vi "扫码枪设置.vi"() -> (2 "确定":bool)   [LabVIEW 2020]
uses:
  Global.vi
  <vilib>/Utility/config.llb/Write Key (String).vi
  <vilib>/Utility/config.llb/NI_LVConfig.lvlib
panel:
  in  "VISA资源名称":refnum<visa-resource-name>="COM5"
  out "error out":errorcluster caption="错误输出"
  in  "error in":errorcluster caption="错误输入（无错误）"
  in  "取消":bool
  in  "连接":bool
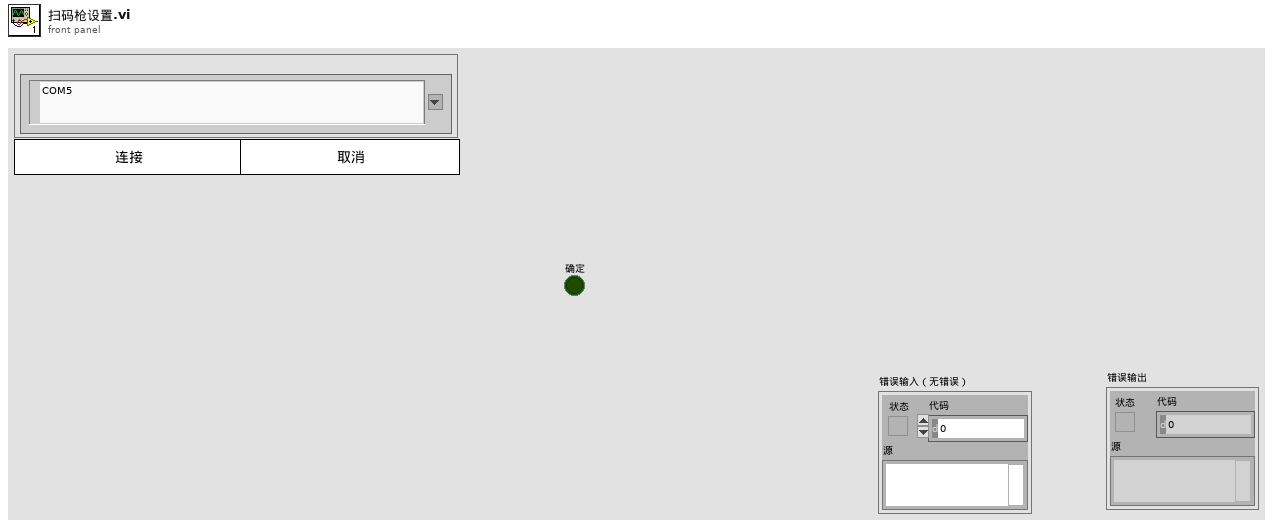
[diagram p1: front panel]
types:
  T1 = typedef "NI_LVConfig.lvlib/Config Data RefNum.ctl" = refnum<k1>
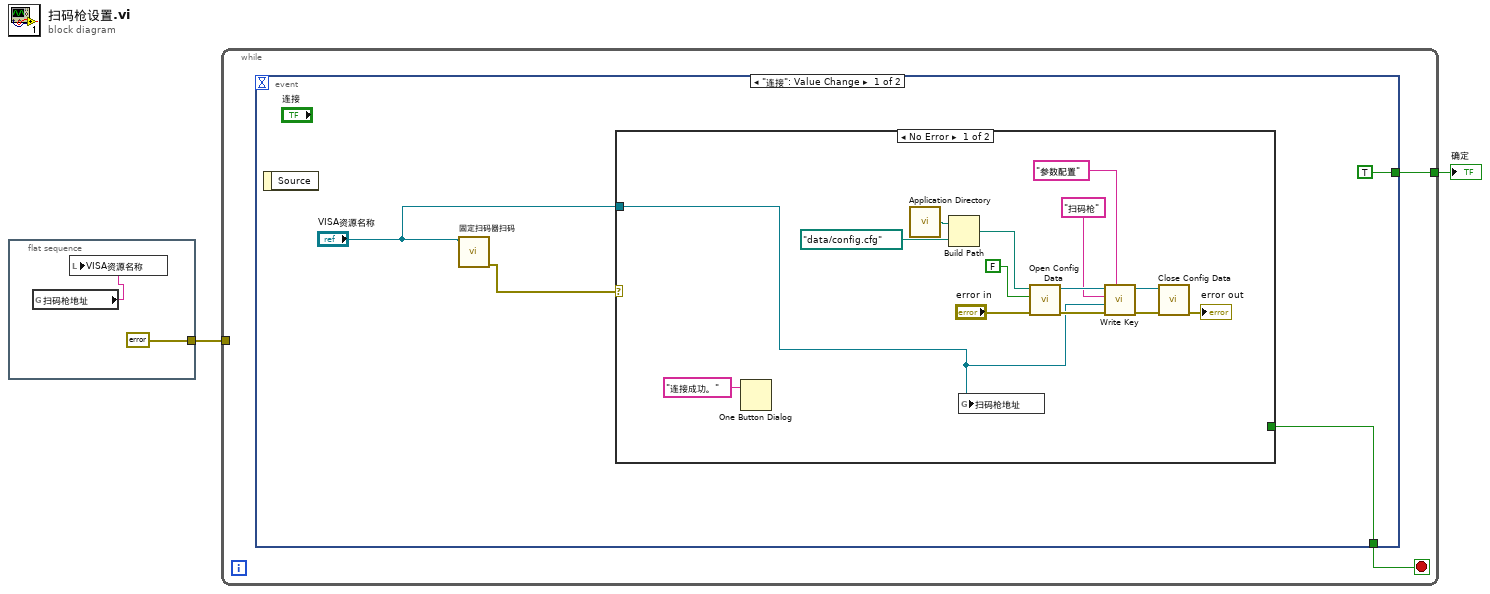
[diagram p0: block diagram]
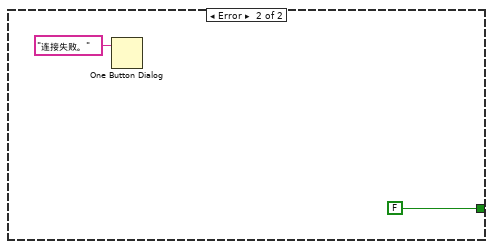
[diagram p2: hidden frame]
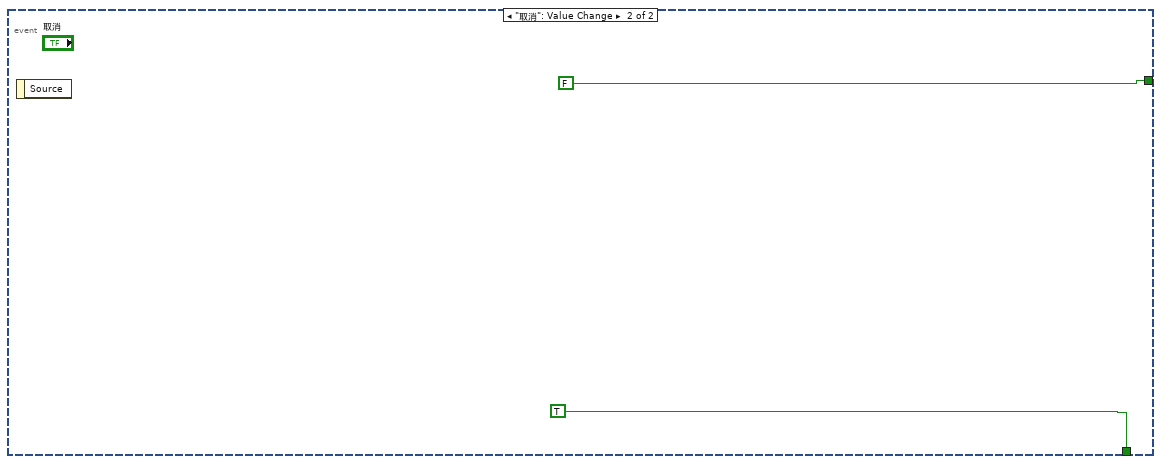
[diagram p3: hidden frame]
diagram:
  n1 = flat-sequence {
    tunnel: [errorcluster {"status"=FALSE, "code"=0, "source"=""} ("错误常量")] -> w1
    frame #0 {
      n2 = global read "Global.vi" "扫码枪地址"() -> (w3:string)
      n3 = local write "VISA资源名称"(w3) -> ()
    }
  }
  n4 = while {
    tunnel: [w5] -> w2
    tunnel: w1 -> [_]
    stop <- w6 stop-if-true
    n5 = event shown="[0] \"连接\": Value Change" {
      selector: _ -> [_ _]
      dyn-events: _ -> [_ _]
      timeout: _ -> [_ _]
      tunnel: [w7 TRUE] -> w6
      tunnel: [TRUE FALSE] -> w5
      event "连接": Value Change {
        n6 = event-data() -> ()  [unwired: 1 in, 1 out]
        n7 = call "固定扫码器扫码.vi"("VISA资源名称"="VISA资源名称") -> ("error out"=w8:errorcluster)  [unwired: 9 in, 1 out]
        n8 = case shown="No Error" w8 {
          tunnel: "VISA资源名称" -> [w12 _]
          tunnel: [_ FALSE] -> w7
          frame No Error {
            n9 = One Button Dialog(message="连接成功。") -> ()  [unwired: 1 in, 1 out]
            n10 = call <vilib>:"Application Directory.vi"() -> ("Application Directory"=w17:path)
            n11 = Build Path(base path=w17, name or relative path=path "data/config.cfg") -> (appended path=w18:path)
            n12 = global write "Global.vi" "扫码枪地址"(w12) -> ()
            n13 = call <vilib>:"Open Config Data.vi"("error in (no error)"="error in", "create file if necessary (T)"=FALSE, "configuration file path"=w18) -> ("error out"=w21:errorcluster, "refnum"=w20:T1)  [unwired: 6 in, 1 out]
            n14 = call-poly <vilib>:"Write Key.vi"("section"="参数配置", "error in (no error)"=w21, "value"=w12, "key"="扫码枪" ("section"), "refnum"=w20) -> ("error out"=w23:errorcluster, "refnum out"=w22:T1)  [unwired: 4 in, 1 out]
            n15 = call <vilib>:"Close Config Data.vi"("error in (no error)"=w23, "refnum"=w22) -> ("error out"=→"error out":errorcluster)  [unwired: 8 in, 1 out]
          }
          frame Error {
            n16 = One Button Dialog(message="连接失败。") -> ()  [unwired: 1 in, 1 out]
          }
        }
      }
      event "取消": Value Change {
        n17 = event-data() -> ()  [unwired: 1 in, 1 out]
      }
    }
  }
  "确定" <- w2
